vi "Send Update Generator Parameter.vi"(7 "Message Priority (Normal)":T4=enum."Normal", 8 "error in (no error)":errorcluster, 10 "Generator Parameters":T1, 11 "Message Enqueuer":refnum<class "Message Enqueuer.lvclass">) -> (0 "error out":errorcluster, 3 "Message Enqueuer out":refnum<class "Message Enqueuer.lvclass">)   [LabVIEW 2016, in "Optimization Framework.lvlib" / "Update Generator Parameter Msg.lvclass"]
doc: "This VI sends the message to an actor."
uses:
  Update Generator Parameter Msg.lvclass
  <vilib>/ActorFramework/Message Enqueuer/Message Enqueuer.lvclass
  <vilib>/ActorFramework/Message Enqueuer/Message Priority.ctl
  Optimization/Controls/Optimization Parameters Generator.ctl
  Master Controller Core/Master Controller/Controls/Current Status.ctl
  Optimization/Controls/Device Control Capabilities.ctl
  C:/Program Files (x86)/National Instruments/LabVIEW 2016/vi.lib/ActorFramework/Message/Message.lvclass
  Update Generator Parameter Msg.lvclass/Update Generator Parameter Msg.ctl
  <vilib>/ActorFramework/Message Enqueuer/Message Enqueuer.lvclass/Message Enqueuer.ctl
  <vilib>/ActorFramework/Message Priority Queue/Priority Enqueue.vi
  Master Controller Core/Master Controller/Master Controller.lvclass
  Optimization/Optimization.lvclass
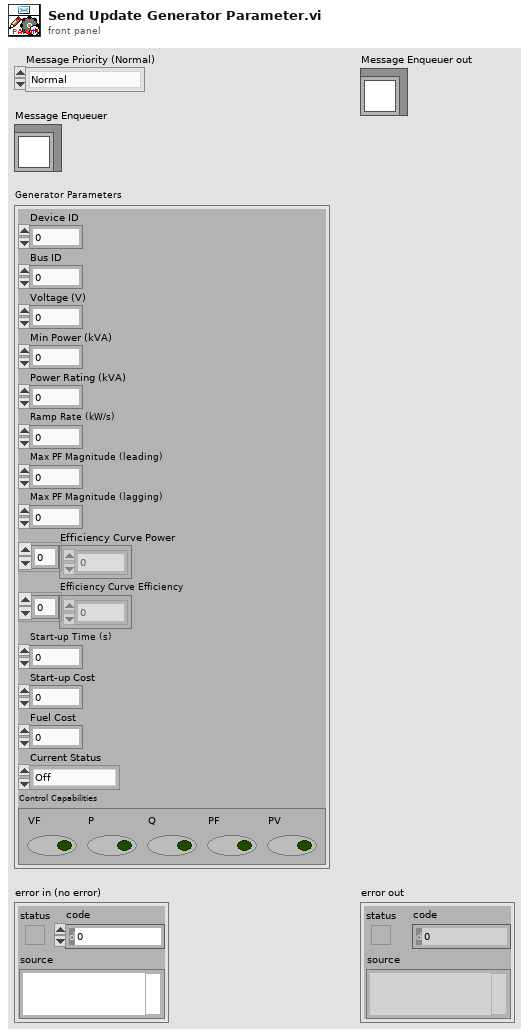
[diagram p1: front panel]
types:
  T1 = typedef "Optimization Framework.lvlib/Optimization.lvclass/Optimization Parameters Generator.ctl" = cluster{"Device ID ":u64, "Bus ID":u16, "Voltage (V)":dbl, "Min Power (kVA)":dbl, "Power Rating (kVA)":dbl, "Ramp Rate (kW/s)":dbl, "Max PF Magnitude (leading)":dbl, "Max PF Magnitude (lagging)":dbl, "Efficiency Curve Power":dbl[], "Efficiency Curve Efficiency":dbl[], "Start-up Time (s)":dbl, "Start-up Cost":dbl, "Fuel Cost":dbl, "Current Status":T2, "Control Capabilities":T3}
  T2 = typedef "Master Controller Core.lvlib/Master Controller.lvclass/Current Status.ctl" = enum8{"Off", "On"}
  T3 = typedef "Optimization Framework.lvlib/Optimization.lvclass/Device Control Capabilities.ctl" = cluster{"VF":bool, "P":bool, "Q":bool, "PF":bool, "PV":bool}
  T4 = typedef "Actor Framework.lvlib/Message Enqueuer.lvclass/Message Priority.ctl" = enum16{"Low", "Normal", "High"}
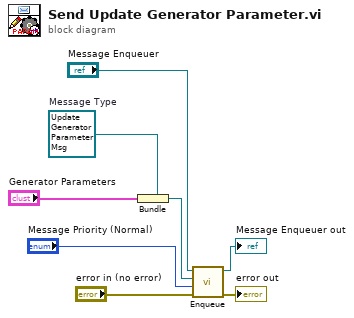
[diagram p0: block diagram]
diagram:
  w5 = refnum<class "Update Generator Parameter Msg.lvclass"> refnum  # Message Type
  n1 = Bundle(cluster=w5, "Generator Parameters") -> (w4:refnum<class "Update Generator Parameter Msg.lvclass">)
  n2 = call <vilib>:"Enqueue.vi"("error in (no error)"="error in (no error)", "Message Priority (Normal)"="Message Priority (Normal)", "Message"=w4, "Message Enqueuer in"="Message Enqueuer") -> ("error out"=→"error out":errorcluster, "Message Enqueuer out"=→"Message Enqueuer out":refnum<class "Message Enqueuer.lvclass">)  [unwired: 6 in]
